vi "PQexec.vi"(8 "error in (no error)":errorcluster, 10 "query":string, 11 "conn":u64) -> (0 "error out":errorcluster, 2 "PGresult":u64, 3 "conn out":u64)   [LabVIEW 2019, in "libpqlv64.lvlib"]
doc: "Submits a command to the server and waits for the result.\nReturns a PGresult pointer or possibly a null pointer. A non-null pointer will generally be returned except in out-of-memory conditions or serious errors such as inability to send the command to the server. If a null pointer is returned, it should be treated like a PGRES_FATAL_ERROR result. Use PQerrorMessage to get more information about such errors.\nhttp://www.postgresql.org/docs/8.3/static/libpq-exec.html"
uses:
  libpqlv64.lvlib
  libpq.dll
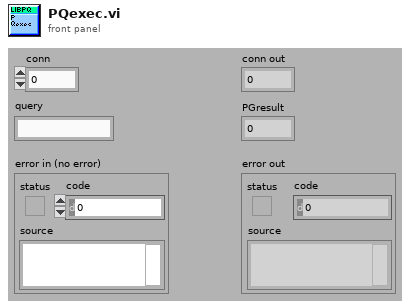
[diagram p1: front panel]
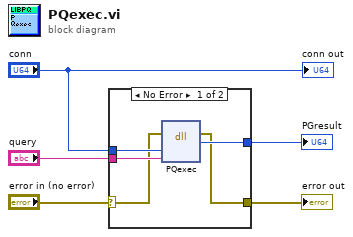
[diagram p0: block diagram]
diagram:
  n1 = case shown="No Error" "error in (no error)" {
    selector: "error in (no error)" -> [w7 w11]
    tunnel: [w6 w11] -> w4
    tunnel: [w10 _] -> w3
    tunnel: "query" -> [w9 _]
    tunnel: "conn" -> [w8 _]
    frame No Error {
      n2 = dll-call lib="libpq.*" fn="PQexec"(error in=w7, "conn"=w8, "query"=w9) -> (error out=w6:errorcluster, "PGresult"=w10:u64)  [unwired: 4 in, 1 out]
    }
    frame Error {
    }
  }
  "PGresult" <- w3
  "error out" <- w4
  "conn out" <- "conn"
